vi "Server.vi"(8 "error in (no error)":errorcluster, 11 "TCP_Server in":refnum<class "TCP_Server.lvclass">) -> (0 "error out":errorcluster, 3 "TCP_Server out":refnum<class "TCP_Server.lvclass">)   [LabVIEW 2013, in "TCP_Server.lvclass"]
uses:
  TCP_Server.lvclass
  TCP_Server.lvclass/TCP_Server.ctl
  LVTM.lvlib
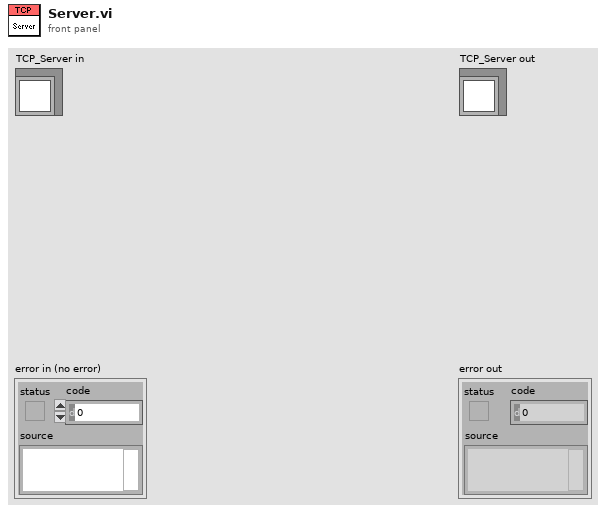
[diagram p1: front panel]
types:
  T1 = cluster{"connection ID":refnum<k5>, "buffer":string}
  T2 = enum16{"Wait for connection", "Connected", "Shutdown"}
  T3 = enum16{"Standard", "Buffered", "CRLF", "Immediate"}
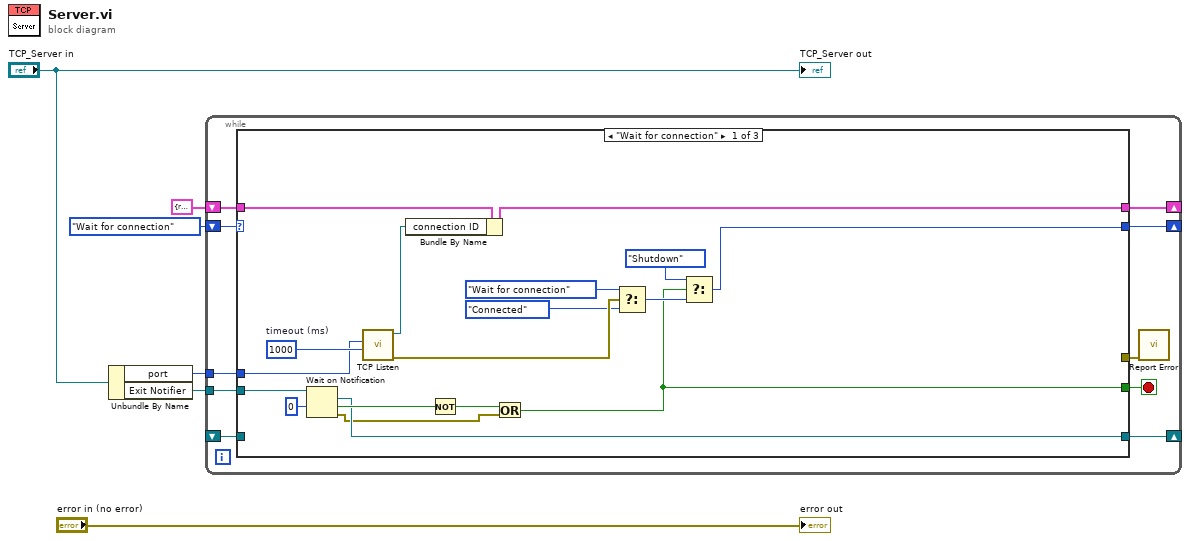
[diagram p0: block diagram]
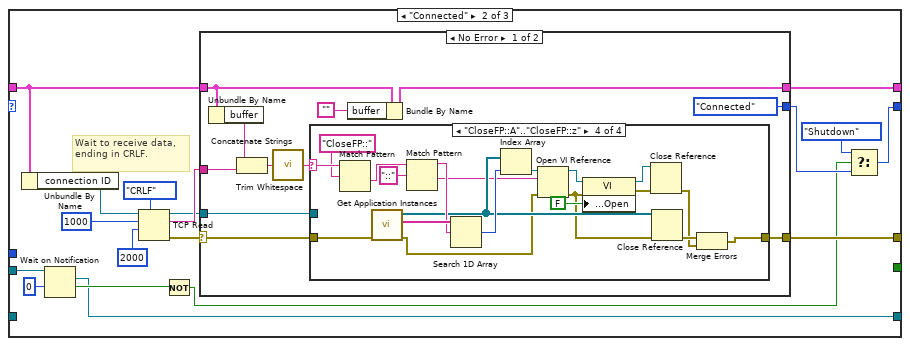
[diagram p2: hidden frame]
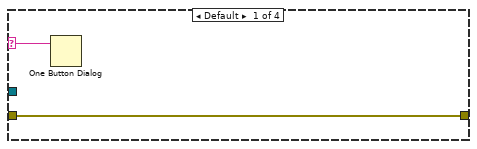
[diagram p3: hidden frame]
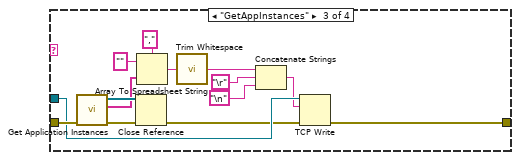
[diagram p5: hidden frame]
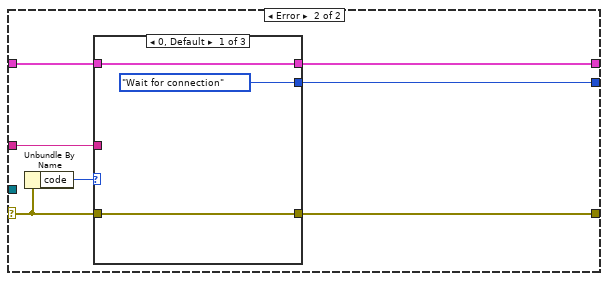
[diagram p6: hidden frame]
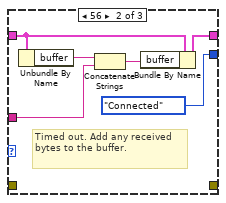
[diagram p7: hidden frame]
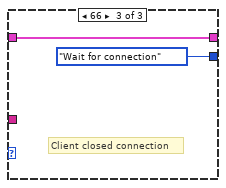
[diagram p8: hidden frame]
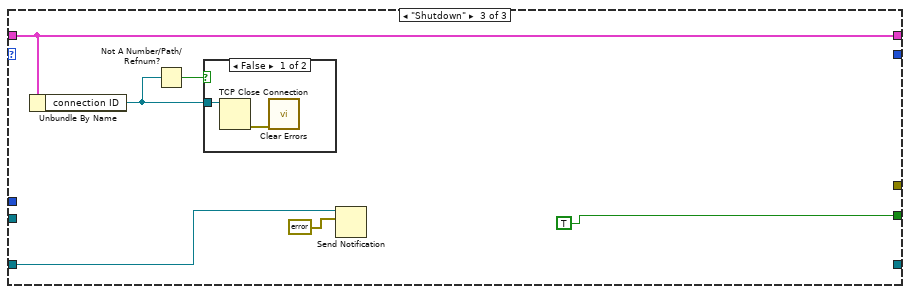
[diagram p9: hidden frame]
diagram:
  n1 = Unbundle By Name("TCP_Server in") -> ("port"=w1:u16, "Exit Notifier"=w2:refnum<notifier>)
  n2 = while {
    shift-right: [w15] -> _
    shift-left: T1 {"connection ID"=refnum, "buffer"=""} -> [w14]
    shift-right: [w13] -> _
    shift-left: T2."Wait for connection" -> [w16]
    tunnel: w2 -> [w11]
    tunnel: w1 -> [w9]
    shift-right: [w8] -> _
    shift-left: _ -> [w7]
    stop <- w12 stop-if-true
    n3 = case shown="\"Wait for connection\"" w16 {
      tunnel: [w33 w43 w124] -> w15
      tunnel: w14 -> [w28 w44 w124]
      tunnel: [_ w46 _] -> w10
      tunnel: [w24 w39 _] -> w13
      tunnel: [w18 _ TRUE] -> w12
      tunnel: w11 -> [w27 w42 _]
      tunnel: w9 -> [w22 _ _]
      tunnel: [w20 w35 _] -> w8
      tunnel: w7 -> [_ _ w122]
      frame "Wait for connection" {
        w34 = 1000  # timeout (ms)
        n4 = Wait on Notification(notifier=w27, timeout in ms (-1)=0) -> (notification=w20:refnum<notifier>, timed out?=w21:bool, error out=w17:errorcluster)  [unwired: 2 in, 1 out]
        n5 = call <vilib>:"TCP Listen.vi"("timeout ms (wait forever: -1)"=w34, "port"=w22) -> ("error out"=w31:errorcluster, "connection ID"=w32:refnum<k5>)  [unwired: 5 in, 3 out]
        n6 = Bundle By Name(cluster=w28, "connection ID"=w32) -> (w33:T1)
        n7 = Not(x=w21) -> (.not. x?=w19:bool)
        n8 = Or(x=w19, y=w17) -> (x .or. y?=w18:bool)
        n9 = Select(t=T2."Wait for connection", s=w31, f=T2."Connected") -> (s? t:f=w25:T2)
        n10 = Select(t=T2."Shutdown", s=w18, f=w25) -> (s? t:f=w24:T2)
      }
      frame "Connected" {
        # "Wait to receive data, ending in CRLF."
        n11 = Unbundle By Name(w44) -> ("connection ID"=w50:refnum<k5>)
        n12 = Wait on Notification(notifier=w42, timeout in ms (-1)=0) -> (notification=w35:refnum<notifier>, timed out?=w37:bool)  [unwired: 2 in, 2 out]
        n13 = TCP Read(connection ID=w50, bytes to read=1000, 7:T3."CRLF" ("mode (standard)"), 9:2000 ("timeout ms (25000)")) -> (connection ID out=w45:refnum<k5>, data out=w48:string, error out=w49:errorcluster)  [unwired: 1 in]
        n14 = Not(x=w37) -> (.not. x?=w36:bool)
        n15 = case shown="No Error" w49 {
          selector: w49 -> [w56 w105]
          tunnel: w48 -> [w62 w101]
          tunnel: [T2."Connected" w104] -> w40
          tunnel: [w55 w106] -> w46
          tunnel: w45 -> [w54 _]
          tunnel: w44 -> [w60 w102]
          tunnel: [w58 w103] -> w43
          frame No Error {
            n16 = Unbundle By Name(w60) -> ("buffer"=w59:string)
            n17 = Concatenate Strings(w59, w62) -> (w61:string)
            n18 = call <vilib>:"Trim Whitespace.vi"("string"=w61) -> ("trimmed string"=w53:string)  [unwired: 1 in]
            n19 = case shown="\"CloseFP::A\"..\"CloseFP::z\"" w53 {
              selector: w53 -> [w65 _ _ w100]
              tunnel: w56 -> [w64 w66 w80 w96]
              tunnel: [w64 w66 w71 w81] -> w55
              tunnel: w54 -> [_ _ w74 _]
              frame Default {
                n20 = One Button Dialog(message=w65) -> ()  [unwired: 1 in, 1 out]
              }
              frame "" {
              }
              frame "GetAppInstances" {
                n21 = call "Get Application Instances.vi"("error in (no error)"=w80) -> ("error out"=w78:errorcluster, "App Instance Names"=w77:string[], "App Instances"=w79:refnum<vi>[])  [unwired: 8 in]
                n22 = Close Reference(reference=w79, error in (no error)=w78) -> (error out=w73:errorcluster)
                n23 = Array To Spreadsheet String(delimiter (Tab)=",", array=w77, 3:"" ("format string")) -> (spreadsheet string=w72:string)
                n24 = call <vilib>:"Trim Whitespace.vi"("string"=w72) -> ("trimmed string"=w70:string)  [unwired: 1 in]
                n25 = Concatenate Strings(w70, "\r", "\n") -> (w69:string)
                n26 = TCP Write(connection ID=w74, data in=w69, error in (no error)=w73) -> (error out=w71:errorcluster)  [unwired: 1 in, 2 out]
              }
              frame "CloseFP::A".."CloseFP::z" {
                n27 = Match Pattern(string=w100, regular expression="CloseFP::") -> (after substring=w97:string)  [unwired: 1 in, 3 out]
                n28 = call "Get Application Instances.vi"("error in (no error)"=w96) -> ("error out"=w89:errorcluster, "App Instance Names"=w95:string[], "App Instances"=w92:refnum<vi>[])  [unwired: 8 in]
                n29 = Match Pattern(string=w97, regular expression="::") -> (before substring=w94:string, after substring=w90:string)  [unwired: 1 in, 2 out]
                n30 = Search 1D Array(1D array=w95, element=w94) -> (index of element=w93:i32)  [unwired: 1 in]
                n31 = Index Array(array=w92, index=w93) -> (element=w91:refnum<vi>)
                n32 = Open VI Reference(application reference (local)=w91, vi path=w90, error in (no error)=w89) -> (vi reference=w85:refnum<vi>, error out=w84:errorcluster)  [unwired: 3 in]
                n33 = property class="VI"(reference=w85, error in=w84, "Front Panel.Open"=FALSE ("Front Panel Window:Open")) -> (reference out=w87:refnum<vi>, error out=w88:errorcluster)
                n34 = Close Reference(reference=w87, error in (no error)=w88) -> (error out=w82:errorcluster)
                n35 = Close Reference(reference=w92, error in (no error)=w84) -> (error out=w83:errorcluster)
                n36 = Merge Errors(w83, w82) -> (w81:errorcluster)
              }
            }
            n37 = Bundle By Name(cluster=w60, "buffer"="") -> (w58:T1)
          }
          frame Error {
            n38 = Unbundle By Name(w105) -> ("code"=w107:i32)
            n39 = case shown="0, Default" w107 {
              tunnel: [w110 _ _] -> w106
              tunnel: w105 -> [w110 _ _]
              tunnel: [T2."Wait for connection" T2."Connected" T2."Wait for connection"] -> w104
              tunnel: [w108 w115 w117] -> w103
              tunnel: w102 -> [w108 w114 w117]
              tunnel: w101 -> [_ w111 _]
              frame 0, Default {
              }
              frame 56 {
                # "Timed out. Add any received bytes to the buffer."
                n40 = Unbundle By Name(w114) -> ("buffer"=w113:string)
                n41 = Concatenate Strings(w113, w111) -> (w112:string)
                n42 = Bundle By Name(cluster=w114, "buffer"=w112) -> (w115:T1)
              }
              frame 66 {
                # "Client closed connection"
              }
            }
          }
        }
        n43 = Select(t=T2."Shutdown", s=w36, f=w40) -> (s? t:f=w39:T2)
      }
      frame "Shutdown" {
        n44 = Unbundle By Name(w124) -> ("connection ID"=w120:refnum<k5>)
        n45 = Not A Number/Path/Refnum?(number/path/refnum=w120) -> (NaN/Path/Refnum?=w119:bool)
        n46 = case shown="False" w119 {
          tunnel: w120 -> [w125 _]
          frame False {
            n47 = TCP Close Connection(connection ID=w125) -> (error out=w126:errorcluster)  [unwired: 1 in, 2 out]
            n48 = call <vilib>:"Clear Errors.vi"("error in (no error)"=w126) -> ()  [unwired: 6 in, 1 out]
          }
          frame True {
          }
        }
        n49 = Send Notification(notification=errorcluster {"status"=FALSE, "code"=0, "source"=""}, notifier=w122) -> ()  [unwired: 1 in, 2 out]
      }
    }
    n50 = call "Report Error.vi"("error in"=w10) -> ()  [unwired: 10 in, 1 out]
  }
  "error out" <- "error in (no error)"
  "TCP_Server out" <- "TCP_Server in"
